vi "Interprocess AI task names to queue names.vi"(11 "Accessors:AI TaskNames*":string[](array[string])) -> (1 "LogEngine Queues":string[](array[string]), 2 "App Queues":string[](array[string]), 3 "All Queues":string[](array[string]))   [LabVIEW 2017, in "DAQ.lvclass"]
doc: "Developed by Kevin Thompson\nkevin@thompsonengineering.net\n\nCopyright 2018-2020\nThompson Engineering, LLC"
uses:
  DAQ.lvclass
  DataTypes/TD AI RawDataQ SelectType--enum.ctl
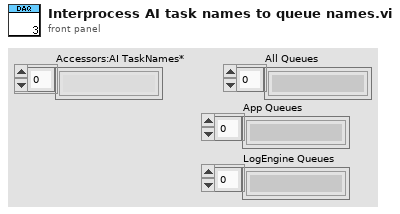
[diagram p1: front panel]
types:
  T1 = typedef "DAQ.lvclass/TD AI RawDataQ SelectType--enum.ctl" = enum16{"InterProcess", "LocalDAQThread"}
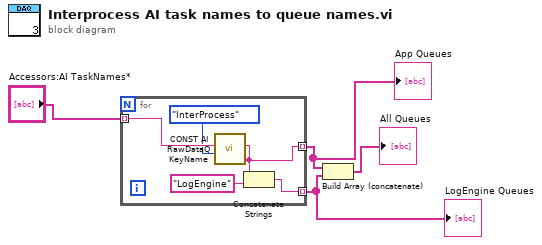
[diagram p0: block diagram]
diagram:
  n1 = for {
    tunnel: "Accessors:AI TaskNames*" -> [w9] mode=indexing
    tunnel: [w6] -> w1 mode=indexing
    tunnel: [w5] -> w2 mode=indexing
    n2 = call "CONST AI RawDataQ KeyName.vi"("Select"=TD_AI_RawDataQ_SelectType--enum."InterProcess", "AI TaskName"=w9) -> ("AI RawDataQ (KeyName)"=w6:string)  [unwired: 9 in]
    n3 = Concatenate Strings(w6, "LogEngine" ("string")) -> (w5:string)
  }
  "App Queues" <- w1
  "LogEngine Queues" <- w2
  n4 = Build Array (concatenate)(w1, w2) -> (→"All Queues":string[])
